vi "Process.vi"(0 "reference in":refnum<class "Battery.lvclass">, 5 "error in":errorcluster) -> (14 "reference out":refnum<class "Battery.lvclass">, 19 "error out":errorcluster)   [LabVIEW 2023, in "Battery.lvclass"]
uses:
  Battery.lvclass
  Model Parameters.ctl
  Simulation Parameters.ctl
  Battery.lvclass/Battery.ctl
  <vilib>/Utility/SystemLogging/NI_SystemLogging.lvlib
panel:
  in  "Battery Tab Control":enum32{"PARAM", "MODEL", "SIMULATION"}(tab)
  in  "Simulation Parameters":T1={"num_rc_pairs"=1, "R0"=0.0015, "R1"=0.001, "C1"=2500.0, "R2"=0.0008, "C2"=40000.0, " nominal_capacity_Ah"=5.0, "upper_voltage_cutoff"=4.2, "lower_voltage_cutoff"=3.0} {"lower_voltage_cutoff" format="%#_13g"; "upper_voltage_cutoff" format="%#_13g"; "nominal_capacity_Ah" format="%#_13g"; "C2" format="%#_13g"; "R2" format="%#_13g"; "C1" format="%#_13g"; "R1" format="%#_13g"; "R0" format="%#_13g"}
  in  "Model Parameters":T2={"chemistry"="Chen2020", "model_type"="SPMe"}
  out "OCV SOC Curve":cluster{"X":dbl, "Y":dbl}[](graph)
  out "State of Charge %":dbl(slide) caption="State of Charge (%)" scale=0.0..100.0 scale format="%.2g"
  out "Terminal Voltage (V)":dbl format="%#.3g"
  out "Battery Simulation":dbl(graph)
  out "Running Status Log":i32(listbox) caption="TEST SERVER LOG"
  out "Temperature (C)":dbl=25.0 format="%.2g"
  out "error info":errorcluster
  out "Last Command":string
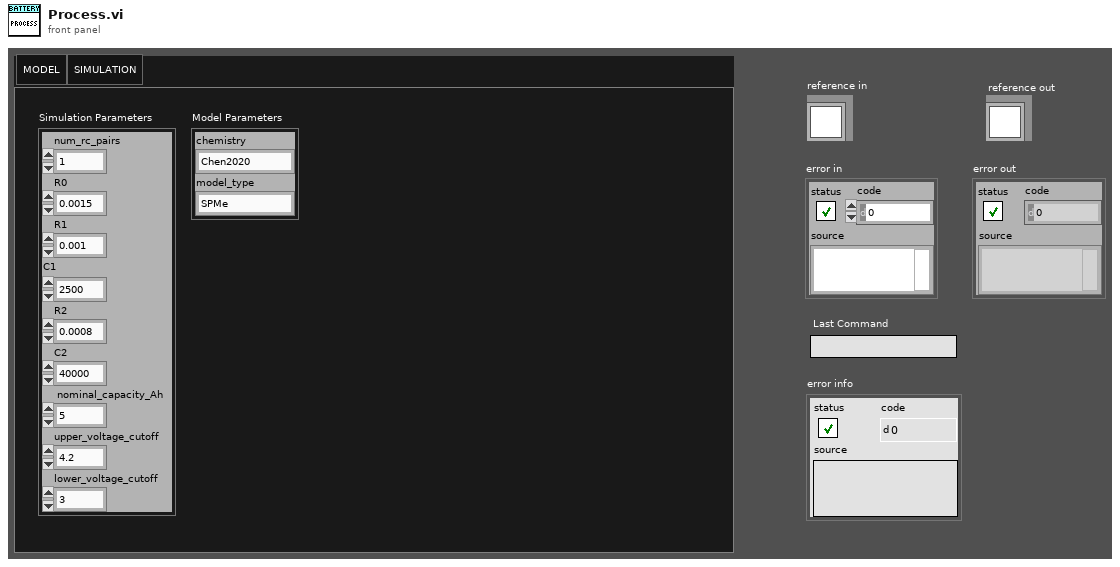
[diagram p1: front panel]
types:
  T1 = typedef "Battery.lvclass/Simulation Parameters.ctl" = cluster{"num_rc_pairs":i32, "R0":dbl, "R1":dbl, "C1":dbl, "R2":dbl, "C2":dbl, " nominal_capacity_Ah":dbl, "upper_voltage_cutoff":dbl, "lower_voltage_cutoff":dbl}
  T2 = typedef "Battery.lvclass/Model Parameters.ctl" = cluster{"chemistry":string, "model_type":string}
  T3 = cluster{"Core":cluster{"Timeout":i32, "Events":cluster{"EventsToProcess":refnum<event-registration>}, "EventFromProcess":refnum<user-event>, "ProcessSyncQueue":refnum<queue>, "QueueFromProcess":refnum<queue>, "Command":string, "Data":variant}}
  T4 = enum32{"Invalid", "Standard", "Closed", "Hidden", "Minimized", "Maximized"}
  T5 = cluster{"EventsToProcess":refnum<event-registration>}
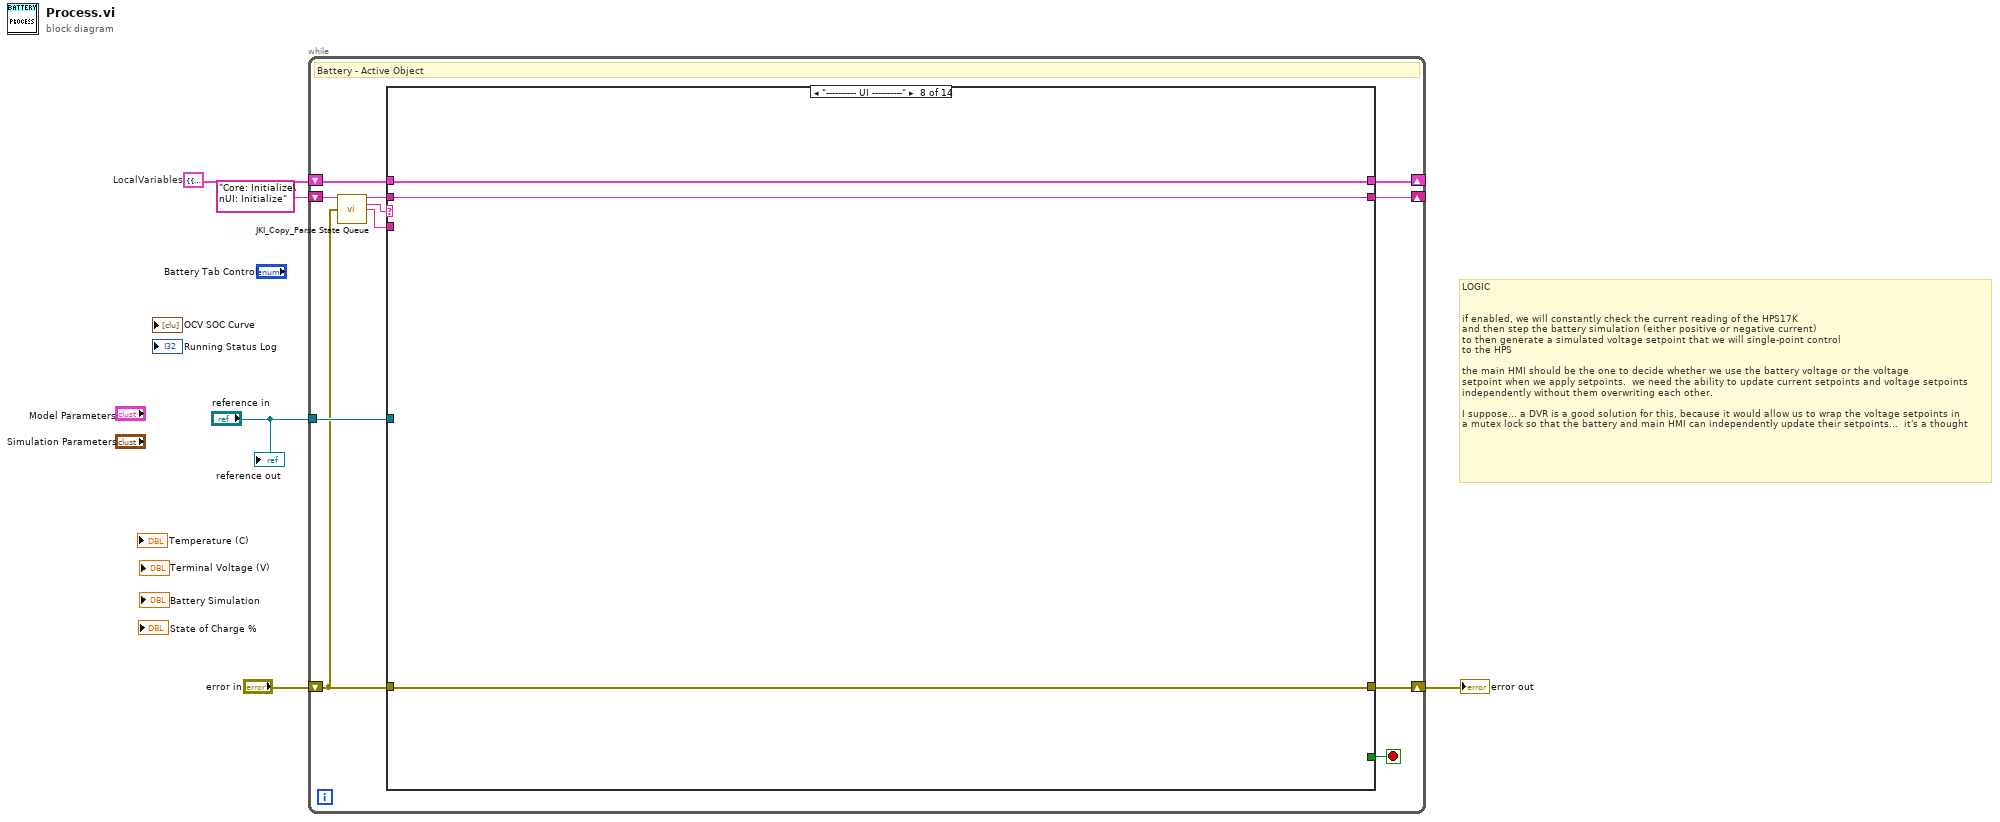
[diagram p0: block diagram]
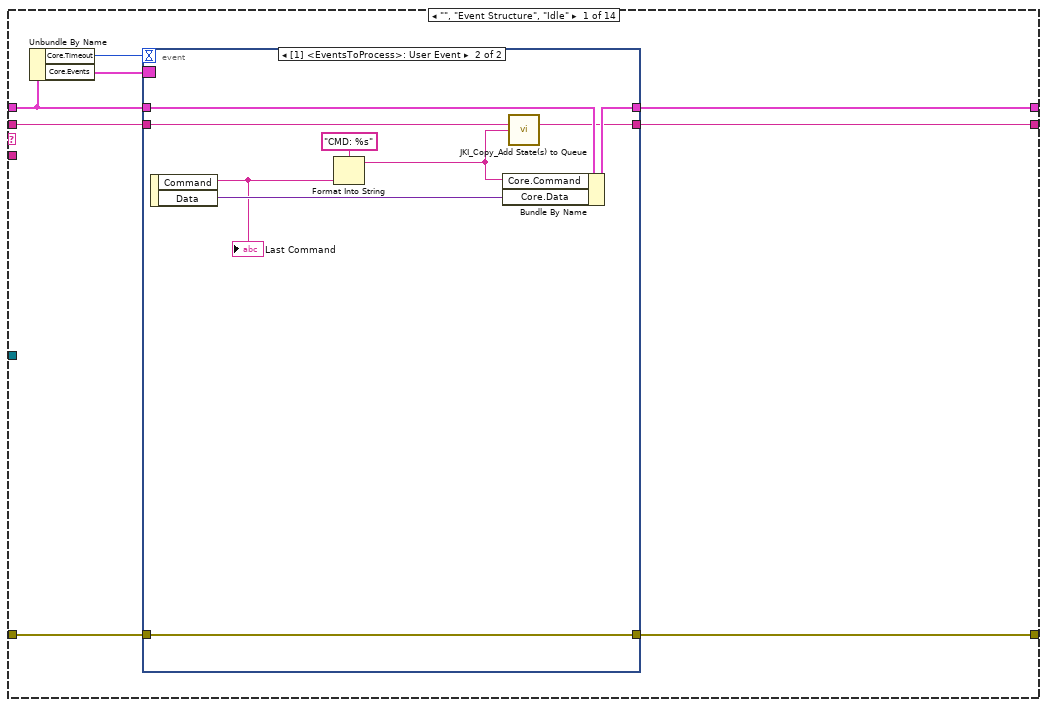
[diagram p2: hidden frame]
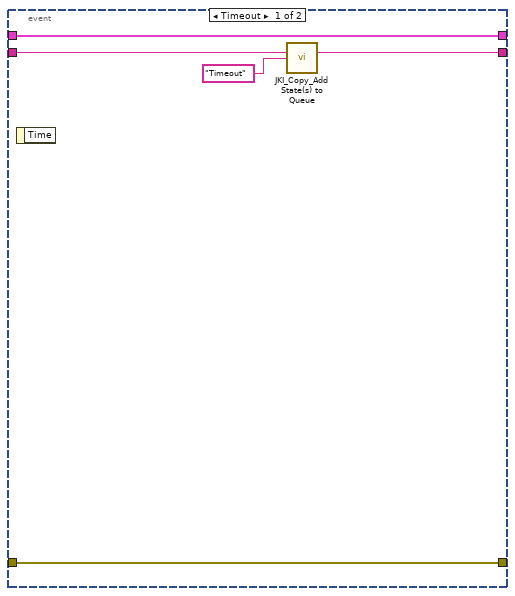
[diagram p3: hidden frame]
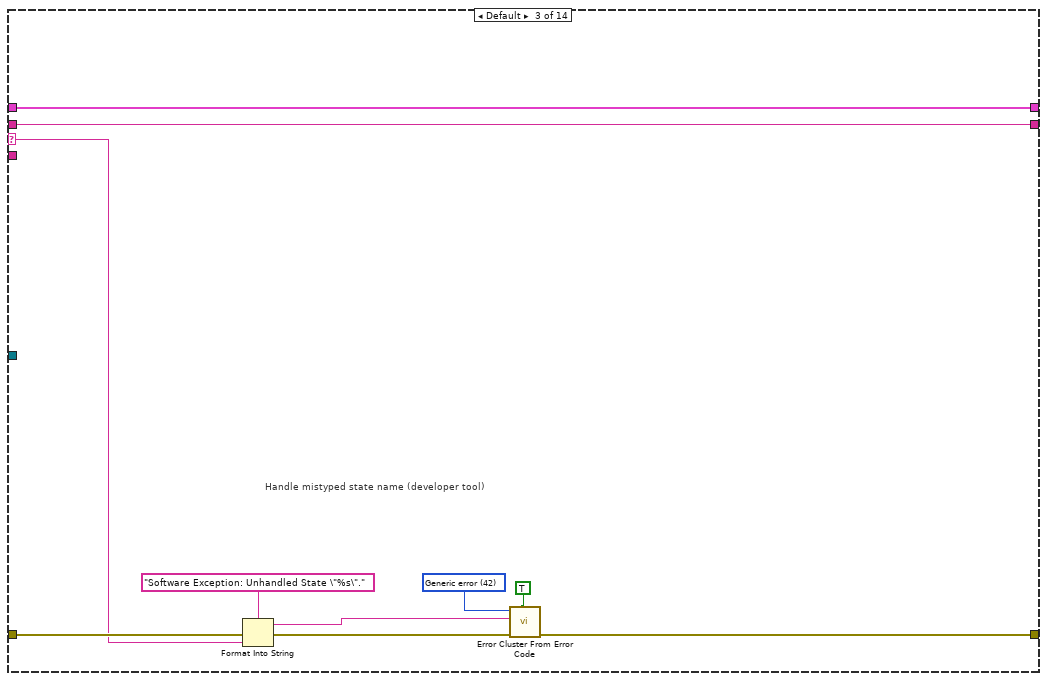
[diagram p5: hidden frame]
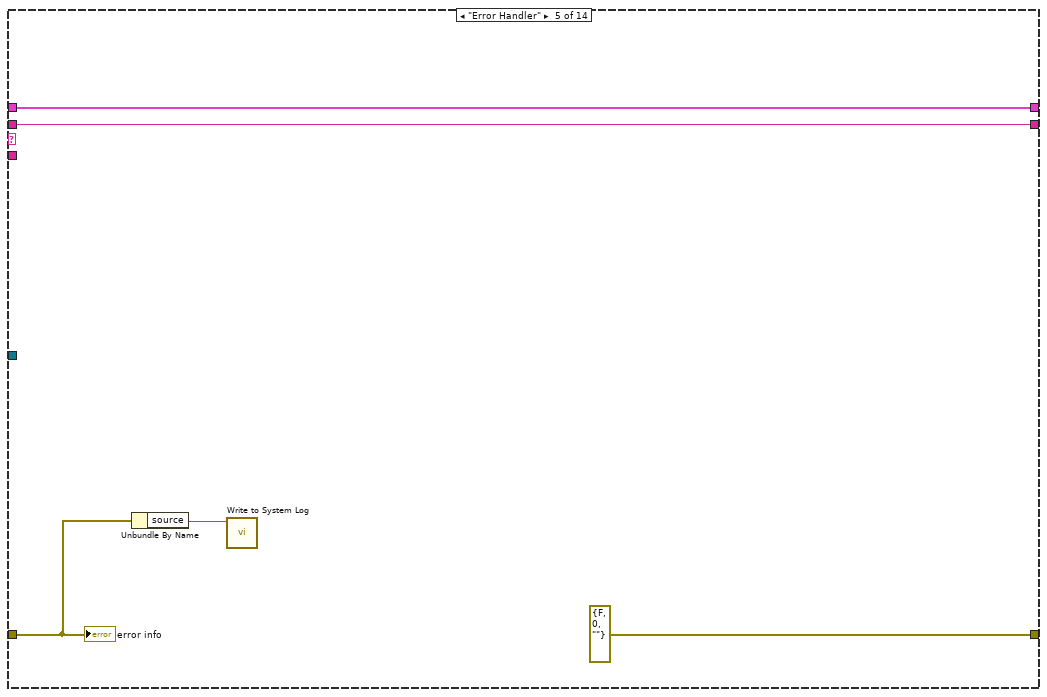
[diagram p7: hidden frame]
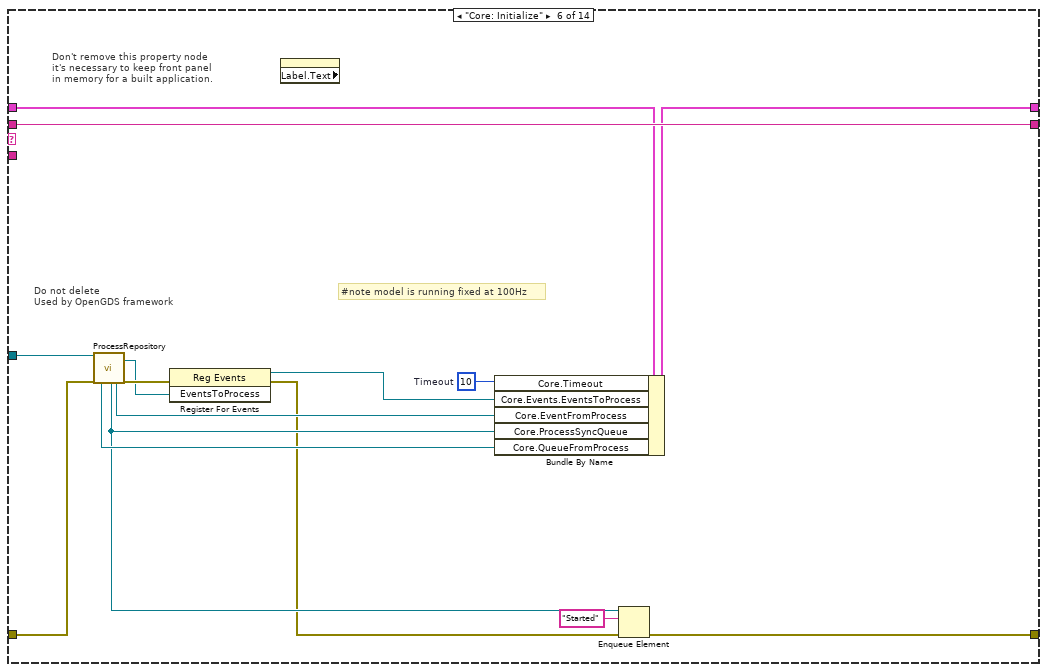
[diagram p8: hidden frame]
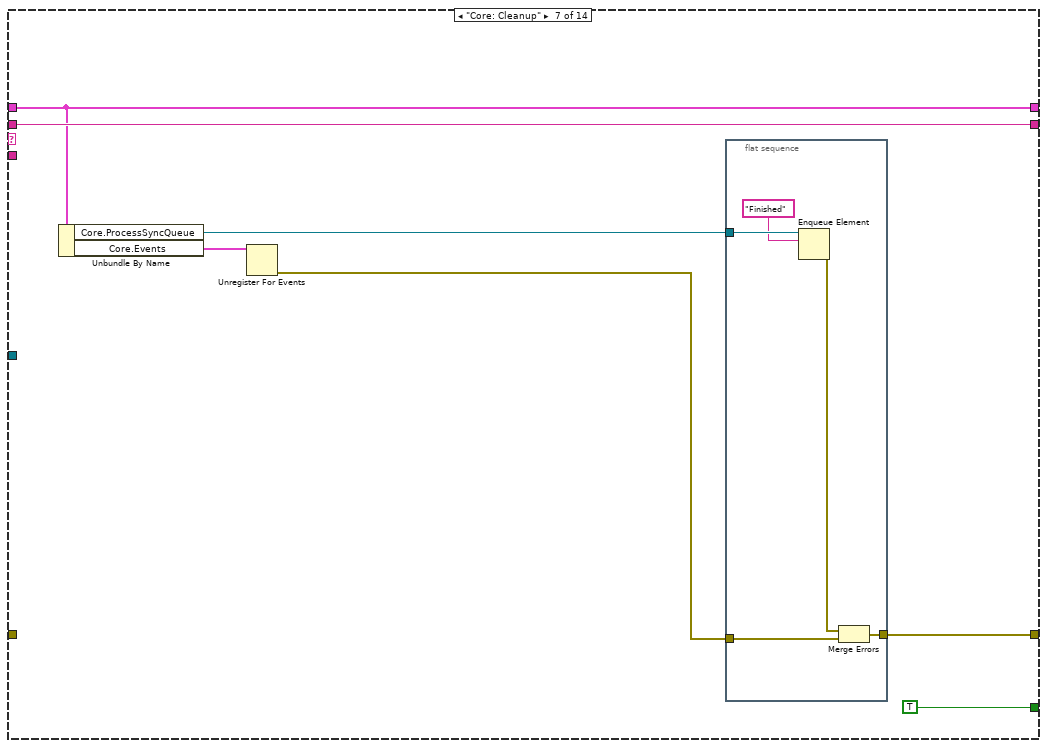
[diagram p9: hidden frame]
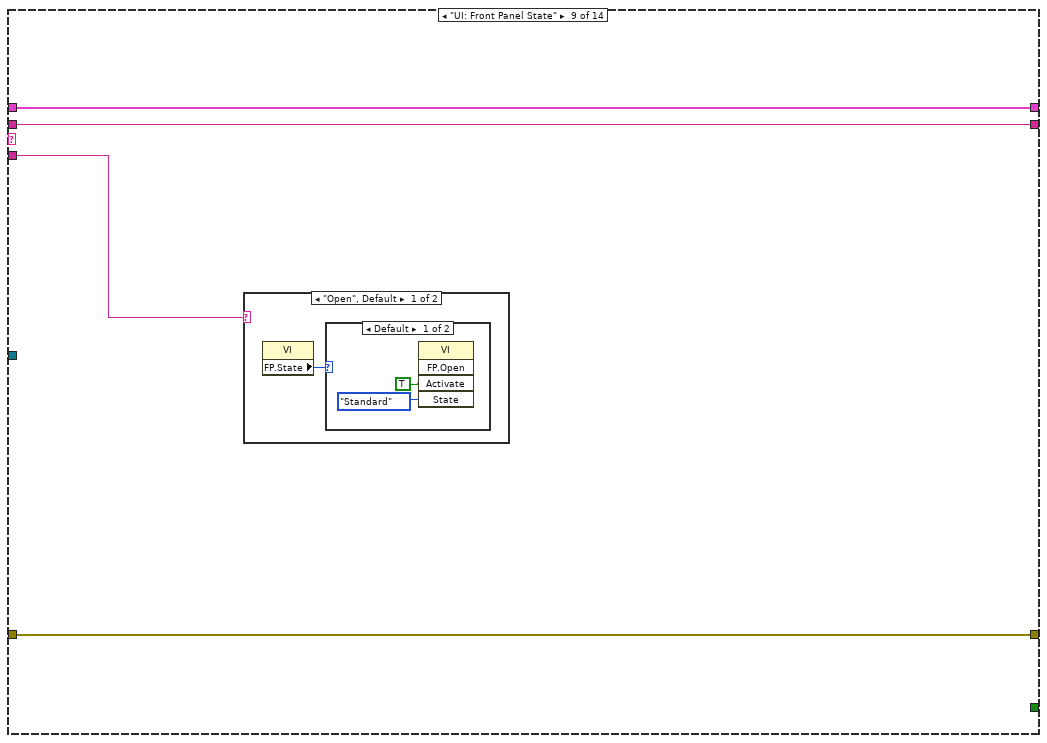
[diagram p10: hidden frame]
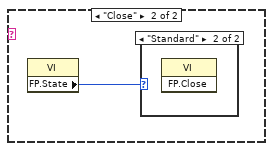
[diagram p12: hidden frame]
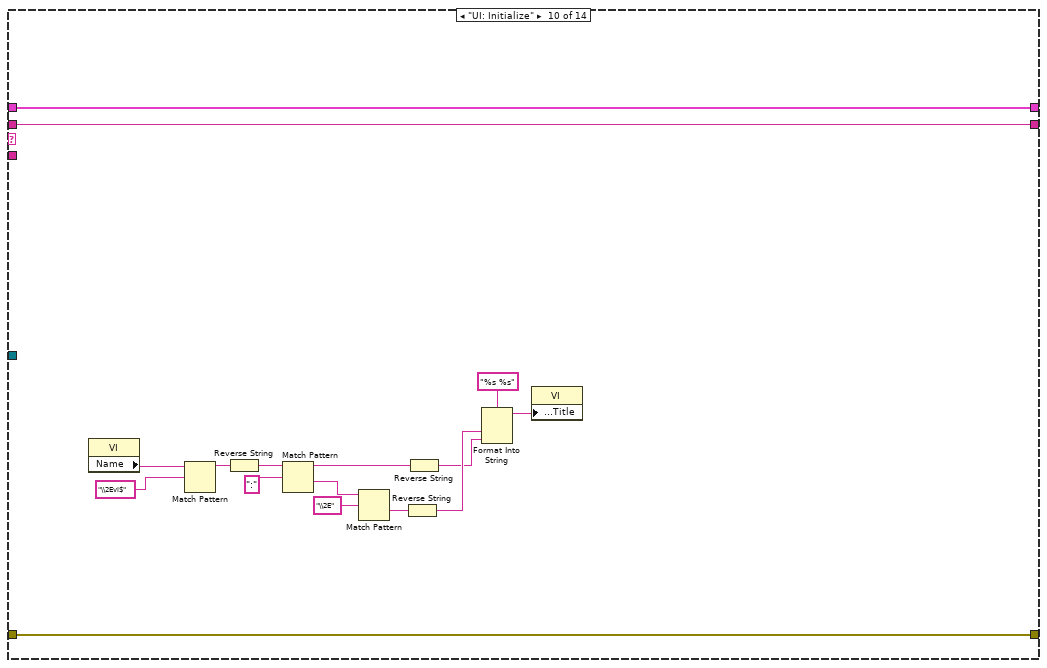
[diagram p14: hidden frame]
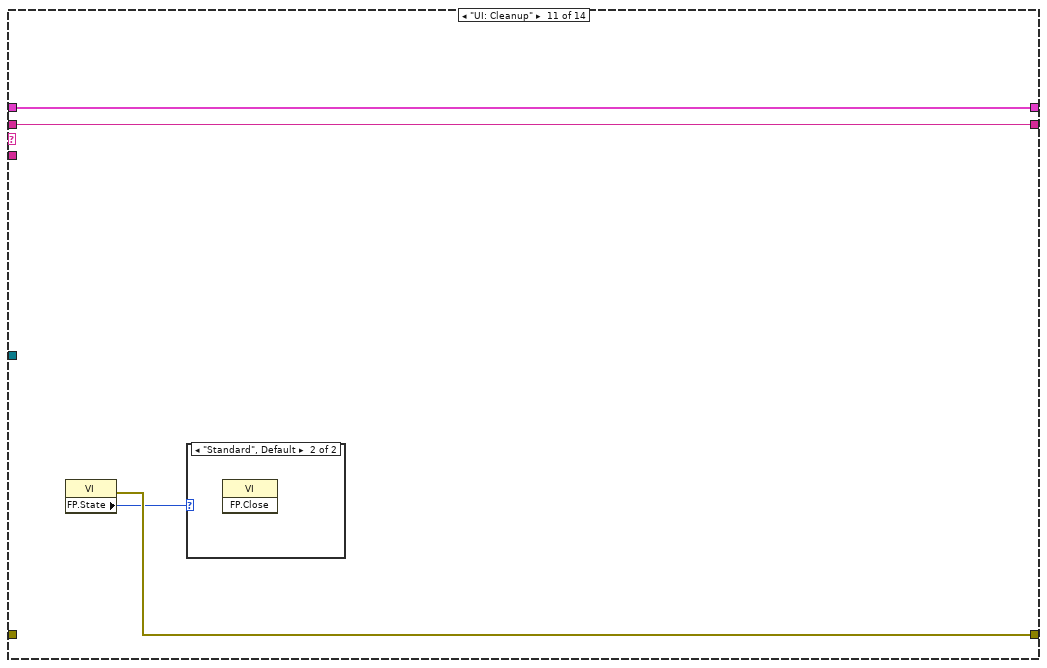
[diagram p15: hidden frame]
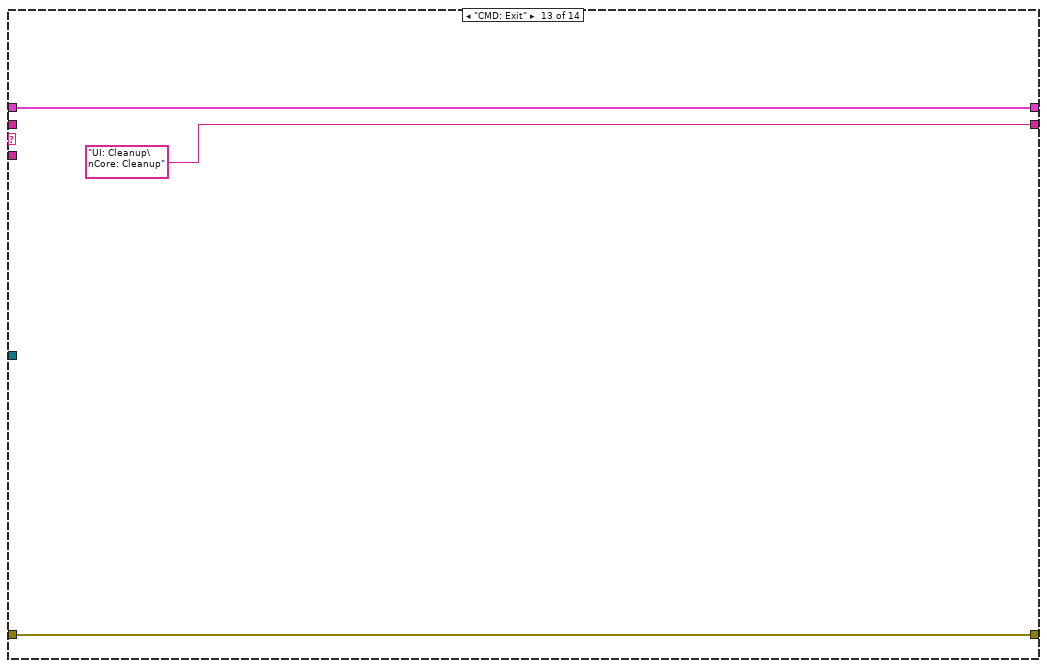
[diagram p18: hidden frame]
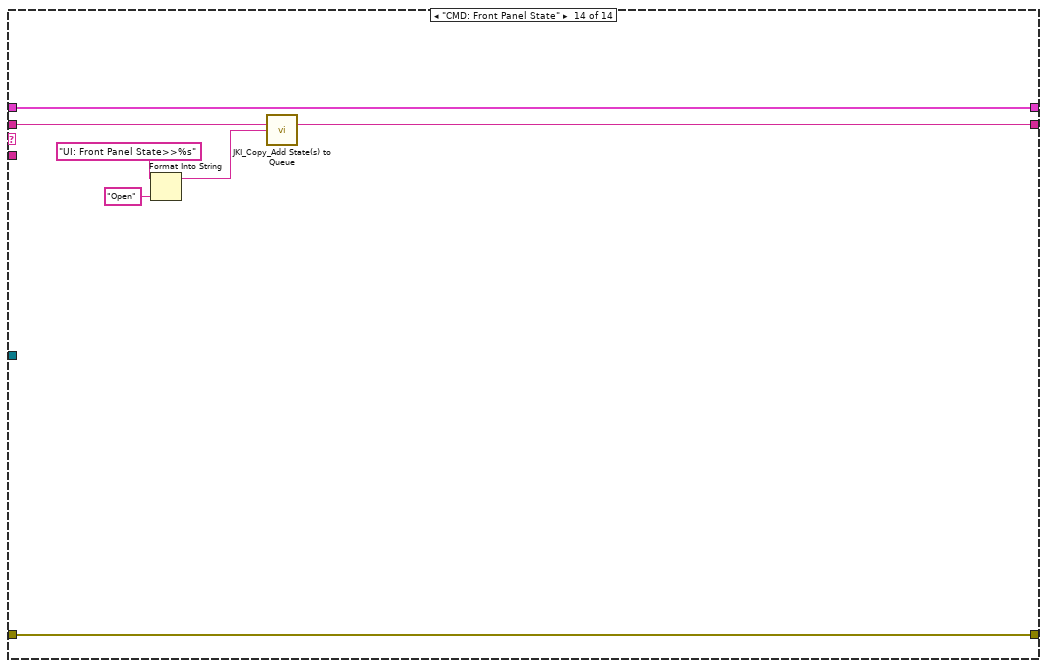
[diagram p19: hidden frame]
diagram:
  w5 = T3 {"Core"={"Timeout"=-1, "Events"={"EventsToProcess"=refnum}, "EventFromProcess"=refnum, "ProcessSyncQueue"=refnum, "QueueFromProcess"=refnum, "Command"="", "Data"=variant}}  # LocalVariables
  # "LOGIC\n\n\nif enabled, we will constantly check the current reading of the HPS17K\nand then step the battery simulation (either positive or negative current) \nto then generate a simulated voltage setpoint that we will single-point control\nto the HPS\n\nthe main HMI should be the one to decide whether we use the battery voltage or the voltage\nsetpoint when we apply setpoints.  we need the ability to update current setpoints and voltage setpoints\nindependently without them overwriting each other.\n\nI suppose... a DVR is a good solution for this, because it would allow us to wrap the voltage setpoints in\na mutex lock so that the battery and main HMI can independently update their setpoints...  it's a thought"
  n1 = while {
    shift-right: [w16] -> w4
    shift-left: "error in" -> [w6]
    shift-right: [w13] -> _
    shift-left: "Core: Initialize\nUI: Initialize" ("States Out") -> [w10]
    shift-right: [w15] -> _
    shift-left: w5 -> [w14]
    tunnel: "reference in" -> [w11]
    stop <- w12 stop-if-true
    # "Battery - Active Object"
    n2 = call <vilib>:"JKI_Copy_Parse State Queue.vi"("State Queue"=w10, "Error In (no error)"=w6) -> ("Remaining States"=w9:string, "Current State"=w7:string, "Arguments"=w8:string)  [unwired: 11 in]
    n3 = case shown="\"---------- UI ----------\"" w7 {
      selector: w7 -> [_ _ w42 _ _ _ _ _ _ _ _ _ _ _]
      tunnel: w6 -> [w18 w41 w44 w52 w58 w60 _ w89 w90 w113 _ w120 w123 w130]
      tunnel: [w19 w41 w43 w52 errorcluster {"status"=FALSE, "code"=0, "source"=""} ("error constant") w74 w77 w89 w90 w113 w115 w120 w123 w130] -> w16
      tunnel: [w24 w40 w51 w53 w59 w72 w78 w88 w92 w111 w116 w119 w122 w129] -> w15
      tunnel: w14 -> [w20 w40 w51 w53 w59 w71 w78 w88 w92 w111 w116 w119 w122 w129]
      tunnel: w9 -> [w22 w39 w50 w54 w56 w73 w81 w87 w93 w112 w117 w118 _ w127]
      tunnel: w8 -> [_ _ _ _ _ _ _ _ w91 _ _ _ _ _]
      tunnel: [w21 w39 w50 w54 w56 w73 w81 w87 w93 w112 w117 w118 "UI: Cleanup\nCore: Cleanup" ("State(s) at Back (\"\")") w125] -> w13
      tunnel: [_ _ _ _ _ _ TRUE _ _ _ _ _ _ _] -> w12
      tunnel: w11 -> [_ _ _ _ _ w61 _ _ _ _ _ _ _ _]
      frame "", "Event Structure", "Idle" {
        n4 = Unbundle By Name(w20) -> ("Core.Timeout"=w17:i32, "Core.Events"=w23:T5)
        n5 = event shown="[1] <EventsToProcess>: User Event" {
          selector: w23 -> [_ _]
          dyn-events: _ -> [_ _]
          timeout: w17 -> [_ _]
          tunnel: w20 -> [w29 w35]
          tunnel: [w29 w38] -> w24
          tunnel: [w26 w30] -> w21
          tunnel: w22 -> [w27 w31]
          tunnel: [w28 w36] -> w19
          tunnel: w18 -> [w28 w36]
          event Timeout {
            n6 = event-data() -> ()  [unwired: 1 in, 1 out]
            n7 = call <vilib>:"JKI_Copy_Add State(s) to Queue.vi"("State(s) in (\"\")"=w27, "State(s) at Back (\"\")"="Timeout" ("State(s) at Back (\"\")")) -> ("States Out"=w26:string)  [unwired: 13 in]
          }
          event User Event {
            n8 = event-data() -> ("Command"=w33:string, "Data"=w37:variant)  [unwired: 1 in]
            "Last Command" <- w33
            n9 = Format Into String(format string="CMD: %s", w33) -> (resulting string=w32:string)  [unwired: 2 in, 1 out]
            n10 = Bundle By Name(cluster=w35, "Core.Command"=w32, "Core.Data"=w37) -> (w38:T3)
            n11 = call <vilib>:"JKI_Copy_Add State(s) to Queue.vi"("State(s) in (\"\")"=w31, "State(s) at Back (\"\")"=w32) -> ("States Out"=w30:string)  [unwired: 13 in]
          }
        }
      }
      frame "---------- Core ----------" {
      }
      frame Default {
        w48 = 42 items=["No error", "Argument error", "Memory is full", "Out of zone", "End of file", "File already open", "Generic file I/O error", "File not found", "File permission error", "Disk is full", "Duplicate path", "Too many files open", "System feature not enabled", "Resource file not found", "Cannot add resource", "Resource not found", "Image not found", "Image memory error", "Pen does not exist", "Config type invalid", "Config token not found", "Config parse error", "Config memory error", "Bad external code format", "Bad external code offset", "External code not present", "Null window", "Destroy window error", "Null menu", "Print aborted", "Bad print record", "Print driver error", "Windows error during printing", "Memory error during printing", "Print dialog error", "Generic print error", "Invalid device refnum", "Device not found", "Device parameter error", "Device unit error", "Cannot open device", "Device call aborted", "Generic error", "Cancelled by user", "Object ID too low", "Object ID too high", "Object not in heap", "Unknown heap", "Unknown object (invalid DefProc)", "Unknown object (DefProc not in table)", "Message out of range", "Invalid (null) method", "Unknown message", "Manager call not supported", "Bad address", "Network operation in progress", "Network operation timed out", "Connection is busy", "Network attribute not supported", "Network error", "Address in use", "System out of memory", "Connection aborted", "Connection refused", "Not connected", "Already connected", "Connection closed", "Initialization error (interapplication manager)", "Bad occurrence", "Wait on unbound occurrence handler", "Occurrence queue overflow", "Datalog type conflict", "Unused", "Unrecognized type (interapplication manager)", "Memory corrupt", "Failed to make temporary DLL", "Old CIN version", "Drag socket not found", "Failed to load drop-object", "Failed to register OLE object", "Failed to release OLE object", "Format specifier type mismatch", "Unknown format specifier", "Too few format specifiers", "Too many format specifiers", "Scan failed", "Newer CIN version", "Error converting to variant", "Runtime menu error", "Password tampered", "Variant attribute not found", "Incompatible variant data type", "Event data is not available", "Event Store is not present", "Occurrence is not found", "Event Queue is not created", "Event info is not available", "Refnum passed is NULL", "Error retrieving Class GUID", "Error retrieving CoClass GUID", "Error retrieving TypeLib GUID.", "Bad built application magic bytes.", "Specific driver is different from the specific driver associated with the Logical Name.", "There is no session opened to the class driver.", "Max Error", "MAX - Error with config objects", "MAX - Error loading configuration", "MAX - Group not supported"]
        # "Handle mistyped state name (developer tool)"
        n12 = Format Into String(format string="Software Exception: Unhandled State \"%s\"." ("message"), error in=w44, w42) -> (resulting string=w47:string, error out=w46:errorcluster)  [unwired: 1 in]
        n13 = call <vilib>:"Error Cluster From Error Code.vi"("show call chain? (False)"=TRUE, "error in (no error)"=w46, "error message (\"\")"=w47, "error code (0)"=w48) -> ("error out"=w43:errorcluster)  [unwired: 5 in]
      }
      frame "Timeout" {
      }
      frame "Error Handler" {
        n14 = Unbundle By Name(w58) -> ("source"=w55:string)
        n15 = call <vilib>:"Write to System Log.vi"("message"=w55) -> ()  [unwired: 10 in, 1 out]
        "error info" <- w58
      }
      frame "Core: Initialize" {
        w62 = 10  # Timeout
        # "#note model is running fixed at 100Hz"
        # "Do not delete\nUsed by OpenGDS framework"
        # "Don't remove this property node\nit's necessary to keep front panel\nin memory for a built application."
        # "Template created by VI Technologies"
        n16 = call "ProcessRepository.vi"("reference in"=w61, "Error In"=w60) -> ("QueueFromProcess"=w66:refnum<queue>, "ProcessSyncQueue"=w64:refnum<queue>, "EventFromProcess"=w67:refnum<user-event>, "EventsToProcess"=w69:refnum<user-event>, "Error Out"=w70:errorcluster)  [unwired: 10 in, 3 out]
        n17 = register-events(error in=w70, w69) -> (reference out=w68:refnum<event-registration>, error out=w63:errorcluster)  [unwired: 1 in]
        n18 = property on="reference in" class="LVClassControl (strict)" props=["Label", "Text"]() -> ()  [unwired: 2 in, 3 out]
        n19 = Bundle By Name(cluster=w71, "Core.Timeout"=w62, "Core.Events.EventsToProcess"=w68, "Core.EventFromProcess"=w67, "Core.ProcessSyncQueue"=w64, "Core.QueueFromProcess"=w66) -> (w72:T3)
        n20 = Enqueue Element(queue=w64, element="Started", error in (no error)=w63) -> (error out=w74:errorcluster)  [unwired: 1 in, 2 out]
      }
      frame "Core: Cleanup" {
        n21 = Unbundle By Name(w78) -> ("Core.ProcessSyncQueue"=w79:refnum<queue>, "Core.Events"=w76:T5)
        n22 = Unregister For Events(event registration refnum=w76) -> (error out=w75:errorcluster)  [unwired: 1 in]
        n23 = flat-sequence {
          tunnel: [w85] -> w77
          tunnel: w79 -> [w84]
          tunnel: w75 -> [w83]
          frame #0 {
            n24 = Enqueue Element(queue=w84, element="Finished") -> (error out=w86:errorcluster)  [unwired: 2 in, 2 out]
            n25 = Merge Errors(w86, w83) -> (w85:errorcluster)
          }
        }
      }
      frame "---------- UI ----------" {
      }
      frame "UI: Front Panel State" {
        n26 = case shown="\"Open\", Default" w91 {
          frame "Open", Default {
            n27 = property class="VI"() -> ("FP.State"=w94:T4)  [unwired: 2 in, 2 out]
            n28 = case shown="Default" w94 {
              frame Default {
                n29 = invoke class="VI" method="FP.Open"("Activate"=TRUE, "State"=T4."Standard") -> ()  [unwired: 3 in, 5 out]
              }
              frame "Standard" {
              }
            }
          }
          frame "Close" {
            n30 = property class="VI"() -> ("FP.State"=w97:T4)  [unwired: 2 in, 2 out]
            n31 = case shown="\"Standard\"" w97 {
              frame Default {
              }
              frame "Standard" {
                n32 = invoke class="VI" method="FP.Close"() -> ()  [unwired: 3 in, 3 out]
              }
            }
          }
        }
      }
      frame "UI: Initialize" {
        n33 = property class="VI"() -> ("Name"=w110:string)  [unwired: 2 in, 2 out]
        n34 = Match Pattern(string=w110, regular expression="\\2Evi$") -> (before substring=w108:string)  [unwired: 1 in, 3 out]
        n35 = Reverse String(1:w108) -> (0:w107:string)
        n36 = Match Pattern(string=w107, regular expression=":") -> (before substring=w105:string, after substring=w104:string)  [unwired: 1 in, 2 out]
        n37 = Match Pattern(string=w104, regular expression="\\2E") -> (after substring=w102:string)  [unwired: 1 in, 3 out]
        n38 = Reverse String(1:w102) -> (0:w101:string)
        n39 = Reverse String(1:w105) -> (0:w100:string)
        n40 = Format Into String(format string="%s %s", w101, w100) -> (resulting string=w99:string)  [unwired: 2 in, 1 out]
        n41 = property class="VI"("Front Panel.Title"=w99) -> ()  [unwired: 2 in, 2 out]
      }
      frame "UI: Cleanup" {
        n42 = property class="VI"() -> (error out=w115:errorcluster, "FP.State"=w114:T4)  [unwired: 2 in, 1 out]
        n43 = case shown="\"Standard\", Default" w114 {
          frame "Closed" {
          }
          frame "Standard", Default {
            n44 = invoke class="VI" method="FP.Close"() -> ()  [unwired: 3 in, 3 out]
          }
        }
      }
      frame "-------- CMD --------" {
      }
      frame "CMD: Exit" {
      }
      frame "CMD: Front Panel State" {
        n45 = Format Into String(format string="UI: Front Panel State>>%s" ("string"), "Open" ("input 1")) -> (resulting string=w126:string)  [unwired: 2 in, 1 out]
        n46 = call <vilib>:"JKI_Copy_Add State(s) to Queue.vi"("State(s) in (\"\")"=w127, "State(s) at Back (\"\")"=w126) -> ("States Out"=w125:string)  [unwired: 13 in]
      }
    }
  }
  "error out" <- w4
  "reference out" <- "reference in"
